vi "AxisNameToID.vi"(10 "MotionPra":T1(array[cluster]), 11 "轴":string[](array[string])) -> (3 "ID":dbl[](array[numeric]), 5 "Size":i32)   [LabVIEW 2017]
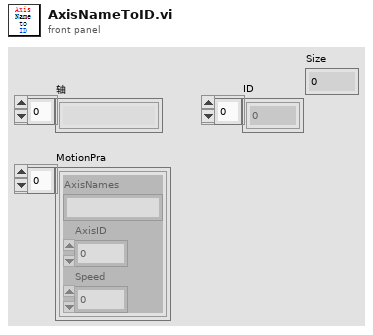
[diagram p1: front panel]
types:
  T1 = cluster{"AxisNames":string, "AxisID":dbl, "Speed":dbl}[]
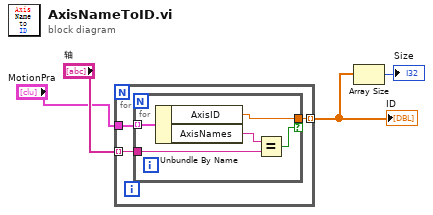
[diagram p0: block diagram]
diagram:
  n1 = for {
    tunnel: "轴" -> [w5] mode=indexing
    tunnel: "MotionPra" -> [w7]
    tunnel: [w6] -> w2 mode=indexing
    n2 = for {
      tunnel: w7 -> [w12] mode=indexing
      tunnel: [w11] -> w6 if=w8
      tunnel: w5 -> [w9]
      n3 = Unbundle By Name(w12) -> ("AxisID"=w11:dbl, "AxisNames"=w10:string)
      n4 = Equal?(x=w10, y=w9) -> (x = y?=w8:bool)
    }
  }
  "ID" <- w2
  n5 = Array Size(array=w2) -> (size(s)=→"Size":i32)
